vi "Escribir_Fichero.vi"(0 "refnum FILE":refnum<file>, 1 "ASIC QR CODE":string, 2 "HORA COMIENZO":timestamp, 5 "OPERADOR":string, 6 "Resultado test":bool, 7 "error in (no error)":errorcluster) -> (20 "refnum out":refnum<file>, 27 "error out":errorcluster)   [LabVIEW 2019]
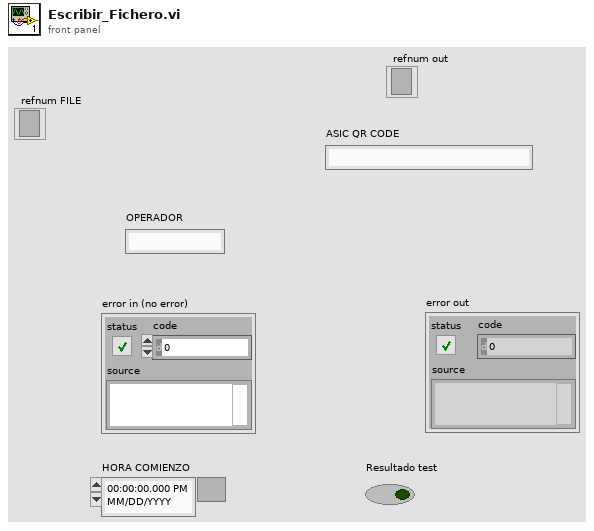
[diagram p1: front panel]
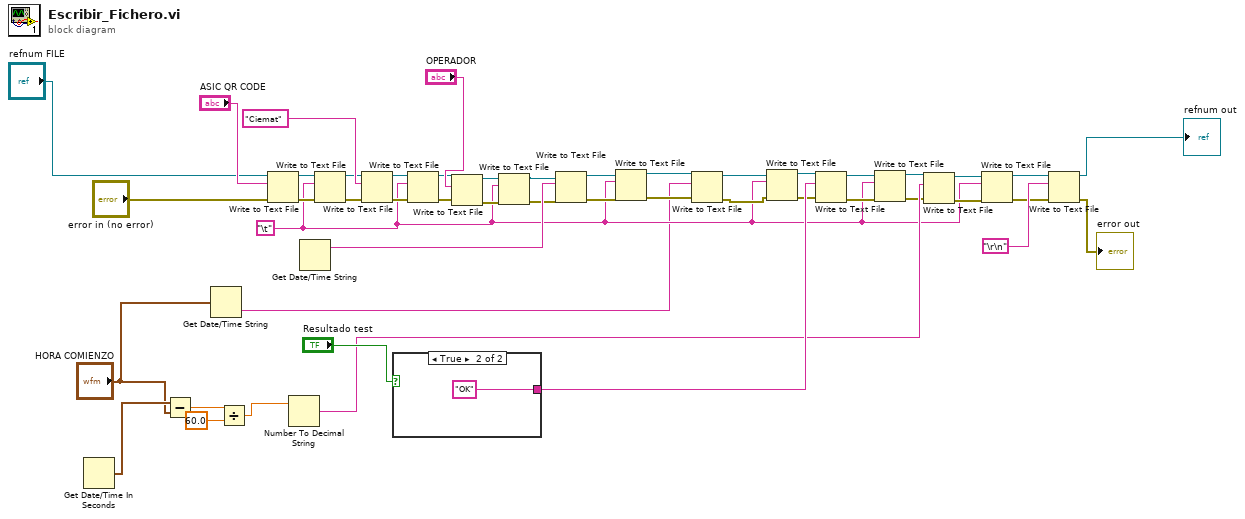
[diagram p0: block diagram]
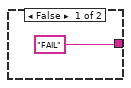
[diagram p2: hidden frame]
diagram:
  w5 = "\t"
  n1 = Get Date/Time In Seconds() -> (seconds since 1Jan1904=w40:timestamp)
  n2 = Subtract(x=w40, y="HORA COMIENZO") -> (x-y=w39:dbl)
  n3 = Get Date/Time String(seconds (now)="HORA COMIENZO") -> (time string=w3:string)  [unwired: 2 in, 1 out]
  n4 = Divide(x=w39, y=60.0) -> (x/y=w37:dbl)
  n5 = Write to Text File(file (use dialog)="refnum FILE", text="ASIC QR CODE", error in="error in (no error)") -> (refnum out=w31:refnum<file>, error out=w30:errorcluster)  [unwired: 1 in, 1 out]
  n6 = Number To Decimal String(number=w37) -> (decimal integer string=w36:string)  [unwired: 1 in]
  n7 = Get Date/Time String() -> (date string=w43:string)  [unwired: 3 in, 1 out]
  n8 = Write to Text File(file (use dialog)=w31, text=w5, error in=w30) -> (refnum out=w29:refnum<file>, error out=w28:errorcluster)  [unwired: 1 in, 1 out]
  n9 = Write to Text File(file (use dialog)=w29, text="Ciemat", error in=w28) -> (refnum out=w27:refnum<file>, error out=w26:errorcluster)  [unwired: 1 in, 1 out]
  n10 = case shown="True" "Resultado test" {
    tunnel: ["FAIL" "OK"] -> w41
    frame False {
    }
    frame True {
    }
  }
  n11 = Write to Text File(file (use dialog)=w27, text=w5, error in=w26) -> (refnum out=w25:refnum<file>, error out=w24:errorcluster)  [unwired: 1 in, 1 out]
  n12 = Write to Text File(file (use dialog)=w25, text="OPERADOR", error in=w24) -> (refnum out=w23:refnum<file>, error out=w22:errorcluster)  [unwired: 1 in, 1 out]
  n13 = Write to Text File(file (use dialog)=w23, text=w5, error in=w22) -> (refnum out=w21:refnum<file>, error out=w20:errorcluster)  [unwired: 1 in, 1 out]
  n14 = Write to Text File(file (use dialog)=w21, text=w43, error in=w20) -> (refnum out=w19:refnum<file>, error out=w18:errorcluster)  [unwired: 1 in, 1 out]
  n15 = Write to Text File(file (use dialog)=w19, text=w5, error in=w18) -> (refnum out=w17:refnum<file>, error out=w16:errorcluster)  [unwired: 1 in, 1 out]
  n16 = Write to Text File(file (use dialog)=w17, text=w3, error in=w16) -> (refnum out=w15:refnum<file>, error out=w14:errorcluster)  [unwired: 1 in, 1 out]
  n17 = Write to Text File(file (use dialog)=w15, text=w5, error in=w14) -> (refnum out=w13:refnum<file>, error out=w12:errorcluster)  [unwired: 1 in, 1 out]
  n18 = Write to Text File(file (use dialog)=w13, text=w41, error in=w12) -> (refnum out=w11:refnum<file>, error out=w10:errorcluster)  [unwired: 1 in, 1 out]
  n19 = Write to Text File(file (use dialog)=w11, text=w5, error in=w10) -> (refnum out=w8:refnum<file>, error out=w9:errorcluster)  [unwired: 1 in, 1 out]
  n20 = Write to Text File(file (use dialog)=w8, text=w36, error in=w9) -> (refnum out=w6:refnum<file>, error out=w7:errorcluster)  [unwired: 1 in, 1 out]
  n21 = Write to Text File(file (use dialog)=w6, text=w5, error in=w7) -> (refnum out=w2:refnum<file>, error out=w1:errorcluster)  [unwired: 1 in, 1 out]
  n22 = Write to Text File(file (use dialog)=w2, text="\r\n", error in=w1) -> (refnum out=→"refnum out":refnum<file>, error out=→"error out":errorcluster)  [unwired: 1 in, 1 out]
